vi "ReadSetting.vi"(5 "FilePath":path) -> (0 "Success":bool, 1 "Setting":T4={"TorqueSensor"={"Interface"="", "Read Unit"=enum."oz.in", "Encoder"=0, "Torque Filter"=0, "Max Torque"=0.0, "Max Power"=0.0, "Max Speed"=0.0, "Scale Factor CW"=0.0, "Scale Factor CCW"=0.0, "Scale Factor Zero"=0.0}, "TorqueSensorL"={"Interface"="", "Read Unit"=enum."Kg.cm", "Encoder"=0, "Torque Filter"=0, "Max Torque"=2.0, "Max Power"=50.0, "Max Speed"=50.0, "Scale Factor CW"=2.0, "Scale Factor CCW"=2.0, "Scale Factor Zero"=2.0}, "Power Meter"={"Wiring"=0, "Interface"="", "1P Mode"=1, "1P CurrentLimit"=0.0, "3P Mode"=1, "3P CurrentLimit"=0.0}, "Thermocouple"={"Interface"="", "value range"="T/C T type -100 ~ 400 degree C", "Channel Count"=8, "Limit 0"=0.0, "Limit 1"=0.0, "Limit 2"=0.0, "Limit 3"=0.0, "Limit 4"=0.0, "Limit 5"=0.0, "Limit 6"=0.0, "Limit 7"=0.0}, "DC-1000"={"Interface"=enum."AD-0"}, "ServoMotor"={"Interface"=enum."AD-0"}, "MotorDriver"={"D_Interface"="", "L_Interface"=""}, "TestMode"=enum."電子中軸測試", "PowerSupply"={"Interface"="", "Current"=50.0, "Voltage"=50.0}} {"Thermocouple"."Limit 7" format="%.1f"; "Thermocouple"."Limit 6" format="%.1f"; "Thermocouple"."Limit 5" format="%.1f"; "Thermocouple"."Limit 4" format="%.1f"; "Thermocouple"."Limit 3" format="%.1f"; "Thermocouple"."Limit 2" format="%.1f"; "Thermocouple"."Limit 1" format="%.1f"; "Thermocouple"."Limit 0" format="%.1f"; "Thermocouple"."Channel Count" min=0 max=24; "Power Meter"."3P Mode" items=["RMS", "MEAN", "DC"]; "Power Meter"."1P Mode" items=["RMS", "MEAN", "DC"]; "Power Meter"."Wiring" items=["AD-0", "AD-1"]; "TorqueSensorL"."Scale Factor Zero" format="%#.6f"; "TorqueSensorL"."Scale Factor CCW" format="%#.6f"; "TorqueSensorL"."Scale Factor CW" format="%#.6f"; "TorqueSensorL"."Torque Filter" items=["OFF", "10Hz", "25Hz", "50Hz", "3Hz", "2Hz", "1Hz"]; "TorqueSensorL"."Encoder" items=["60-ppr"=60, "600-ppr"=600, "6000-ppr"=6000, "8192-ppr"=8192, "20-ppr"=20, "30-ppr"=30, "1-ppr"=1, "2-ppr"=2, "6-ppr"=6]; "TorqueSensor"."Scale Factor Zero" format="%#.6f"; "TorqueSensor"."Scale Factor CCW" format="%#.6f"; "TorqueSensor"."Scale Factor CW" format="%#.6f"; "TorqueSensor"."Torque Filter" items=["OFF", "10Hz", "25Hz", "50Hz", "3Hz", "2Hz", "1Hz"]; "TorqueSensor"."Encoder" items=["60-ppr"=60, "600-ppr"=600, "6000-ppr"=6000, "8192-ppr"=8192, "20-ppr"=20, "30-ppr"=30, "1-ppr"=1, "2-ppr"=2, "6-ppr"=6]}, 2 "RcpFilePath.dup":path)   [LabVIEW 2024]
uses:
  MFActor/SystemSettings.ctl
panel:
  in  "Setting_V4":T1={"TorqueSensor"={"Interface"="", "Read Unit"=enum."Kg.cm", "Encoder"=0, "Torque Filter"=0, "Max Torque"=2.0, "Max Power"=50.0, "Max Speed"=50.0, "Scale Factor CW"=2.0, "Scale Factor CCW"=2.0, "Scale Factor Zero"=2.0}, "TorqueSensorL"={"Interface"="", "Read Unit"=enum."Kg.cm", "Encoder"=0, "Torque Filter"=0, "Max Torque"=2.0, "Max Power"=50.0, "Max Speed"=50.0, "Scale Factor CW"=2.0, "Scale Factor CCW"=2.0, "Scale Factor Zero"=2.0}, "Power Meter"={"Wiring"=0, "Interface"="", "1P Mode"=1, "1P CurrentLimit"=0.0, "3P Mode"=1, "3P CurrentLimit"=0.0}, "Thermocouple"={"Interface"="", "value range"="T/C T type -100 ~ 400 degree C", "Channel Count"=8, "Limit 0"=0.0, "Limit 1"=0.0, "Limit 2"=0.0, "Limit 3"=0.0, "Limit 4"=0.0, "Limit 5"=0.0, "Limit 6"=0.0, "Limit 7"=0.0}, "DC-1000"={"Interface"=enum."AD-1"}, "ServoMotor"={"Interface"=enum."AD-1"}, "MotorDriver"={"D_Interface"="", "L_Interface"=""}, "TestMode"=enum."電子中軸測試", "PowerSupply"={"Interface"="", "Current"=50.0, "Voltage"=50.0}} {"Thermocouple"."Limit 7" format="%.1f"; "Thermocouple"."Limit 6" format="%.1f"; "Thermocouple"."Limit 5" format="%.1f"; "Thermocouple"."Limit 4" format="%.1f"; "Thermocouple"."Limit 3" format="%.1f"; "Thermocouple"."Limit 2" format="%.1f"; "Thermocouple"."Limit 1" format="%.1f"; "Thermocouple"."Limit 0" format="%.1f"; "Thermocouple"."Channel Count" min=0 max=24; "Power Meter"."3P Mode" items=["RMS", "MEAN", "DC"]; "Power Meter"."1P Mode" items=["RMS", "MEAN", "DC"]; "Power Meter"."Wiring" items=["1P2W", "1P2W+3P3W3M"]; "TorqueSensorL"."Scale Factor Zero" format="%#.6f"; "TorqueSensorL"."Scale Factor CCW" format="%#.6f"; "TorqueSensorL"."Scale Factor CW" format="%#.6f"; "TorqueSensorL"."Torque Filter" items=["OFF", "10Hz", "25Hz", "50Hz", "3Hz", "2Hz", "1Hz"]; "TorqueSensorL"."Encoder" items=["60-ppr"=60, "600-ppr"=600, "6000-ppr"=6000, "8192-ppr"=8192, "20-ppr"=20, "30-ppr"=30, "1-ppr"=1, "2-ppr"=2, "6-ppr"=6]; "TorqueSensor"."Scale Factor Zero" format="%#.6f"; "TorqueSensor"."Scale Factor CCW" format="%#.6f"; "TorqueSensor"."Scale Factor CW" format="%#.6f"; "TorqueSensor"."Torque Filter" items=["OFF", "10Hz", "25Hz", "50Hz", "3Hz", "2Hz", "1Hz"]; "TorqueSensor"."Encoder" items=["60-ppr"=60, "600-ppr"=600, "6000-ppr"=6000, "8192-ppr"=8192, "20-ppr"=20, "30-ppr"=30, "1-ppr"=1, "2-ppr"=2, "6-ppr"=6]}
  in  "Setting_V3":T2={"TorqueSensor"={"Interface"="", "Read Unit"=enum."Kg.cm", "Encoder"=0, "Torque Filter"=0, "Max Torque"=2.0, "Max Power"=50.0, "Max Speed"=50.0, "Scale Factor CW"=2.0, "Scale Factor CCW"=2.0, "Scale Factor Zero"=2.0}, "TorqueSensorL"={"Interface"="", "Read Unit"=enum."Kg.cm", "Encoder"=0, "Torque Filter"=0, "Max Torque"=2.0, "Max Power"=50.0, "Max Speed"=50.0, "Scale Factor CW"=2.0, "Scale Factor CCW"=2.0, "Scale Factor Zero"=2.0}, "Power Meter"={"Wiring"=0, "Interface"="", "1P Mode"=1, "1P CurrentLimit"=0.0, "3P Mode"=1, "3P CurrentLimit"=0.0}, "Thermocouple"={"Interface"="", "value range"="T/C T type -100 ~ 400 degree C", "Channel Count"=8, "Limit 0"=0.0, "Limit 1"=0.0, "Limit 2"=0.0, "Limit 3"=0.0, "Limit 4"=0.0, "Limit 5"=0.0, "Limit 6"=0.0, "Limit 7"=0.0}, "DC-1000"={"Interface"=enum."AD-1"}, "ServoMotor"={"Interface"=enum."AD-1"}, "MotorDriver"={"D_Interface"="", "L_Interface"=""}, "TestMode"=enum."電子中軸測試"} {"Thermocouple"."Limit 7" format="%.1f"; "Thermocouple"."Limit 6" format="%.1f"; "Thermocouple"."Limit 5" format="%.1f"; "Thermocouple"."Limit 4" format="%.1f"; "Thermocouple"."Limit 3" format="%.1f"; "Thermocouple"."Limit 2" format="%.1f"; "Thermocouple"."Limit 1" format="%.1f"; "Thermocouple"."Limit 0" format="%.1f"; "Thermocouple"."Channel Count" min=0 max=24; "Power Meter"."3P Mode" items=["RMS", "MEAN", "DC"]; "Power Meter"."1P Mode" items=["RMS", "MEAN", "DC"]; "Power Meter"."Wiring" items=["1P2W", "1P2W+3P3W3M"]; "TorqueSensorL"."Scale Factor Zero" format="%#.6f"; "TorqueSensorL"."Scale Factor CCW" format="%#.6f"; "TorqueSensorL"."Scale Factor CW" format="%#.6f"; "TorqueSensorL"."Torque Filter" items=["OFF", "10Hz", "25Hz", "50Hz", "3Hz", "2Hz", "1Hz"]; "TorqueSensorL"."Encoder" items=["60-ppr"=60, "600-ppr"=600, "6000-ppr"=6000, "8192-ppr"=8192, "20-ppr"=20, "30-ppr"=30, "1-ppr"=1, "2-ppr"=2, "6-ppr"=6]; "TorqueSensor"."Scale Factor Zero" format="%#.6f"; "TorqueSensor"."Scale Factor CCW" format="%#.6f"; "TorqueSensor"."Scale Factor CW" format="%#.6f"; "TorqueSensor"."Torque Filter" items=["OFF", "10Hz", "25Hz", "50Hz", "3Hz", "2Hz", "1Hz"]; "TorqueSensor"."Encoder" items=["60-ppr"=60, "600-ppr"=600, "6000-ppr"=6000, "8192-ppr"=8192, "20-ppr"=20, "30-ppr"=30, "1-ppr"=1, "2-ppr"=2, "6-ppr"=6]}
  in  "Setting_V2":T3={"TorqueSensor"={"Interface"="", "Read Unit"=enum."Kg.cm", "Encoder"=0, "Torque Filter"=0, "Max Torque"=2.0, "Max Power"=50.0, "Max Speed"=50.0, "Scale Factor CW"=2.0, "Scale Factor CCW"=2.0, "Scale Factor Zero"=2.0}, "DC-1000"={"Interface"=enum."AD-1"}, "ServoMotor"={"Interface"=enum."AD-1"}, "MotorDriver"={"D_Interface"="", "L_Interface"=""}, "SwapDL"=FALSE} {"TorqueSensor"."Scale Factor Zero" format="%#.6f"; "TorqueSensor"."Scale Factor CCW" format="%#.6f"; "TorqueSensor"."Scale Factor CW" format="%#.6f"; "TorqueSensor"."Torque Filter" items=["OFF", "10Hz", "25Hz", "50Hz", "3Hz", "2Hz", "1Hz"]; "TorqueSensor"."Encoder" items=["60-ppr"=60, "600-ppr"=600, "6000-ppr"=6000, "8192-ppr"=8192, "20-ppr"=20, "30-ppr"=30, "1-ppr"=1, "2-ppr"=2, "6-ppr"=6]}
  in  "Setting_V1":T5={"TorqueSensor"={"Interface"="", "Read Unit"=enum."Kg.cm", "Encoder"=0, "Torque Filter"=0, "Max Torque"=2.0, "Max Power"=50.0, "Max Speed"=50.0, "Scale Factor CW"=2.0, "Scale Factor CCW"=2.0, "Scale Factor Zero"=2.0}, "DC-1000"={"Interface"=enum."AD-1"}, "ServoMotor"={"Interface"=enum."AD-1"}, "MotorDriver"={"D_Interface"="", "L_Interface"=""}} {"TorqueSensor"."Scale Factor Zero" format="%#.6f"; "TorqueSensor"."Scale Factor CCW" format="%#.6f"; "TorqueSensor"."Scale Factor CW" format="%#.6f"; "TorqueSensor"."Torque Filter" items=["OFF", "10Hz", "25Hz", "50Hz", "3Hz", "2Hz", "1Hz"]; "TorqueSensor"."Encoder" items=["60-ppr"=60, "600-ppr"=600, "6000-ppr"=6000, "8192-ppr"=8192, "20-ppr"=20, "30-ppr"=30, "1-ppr"=1, "2-ppr"=2, "6-ppr"=6]}
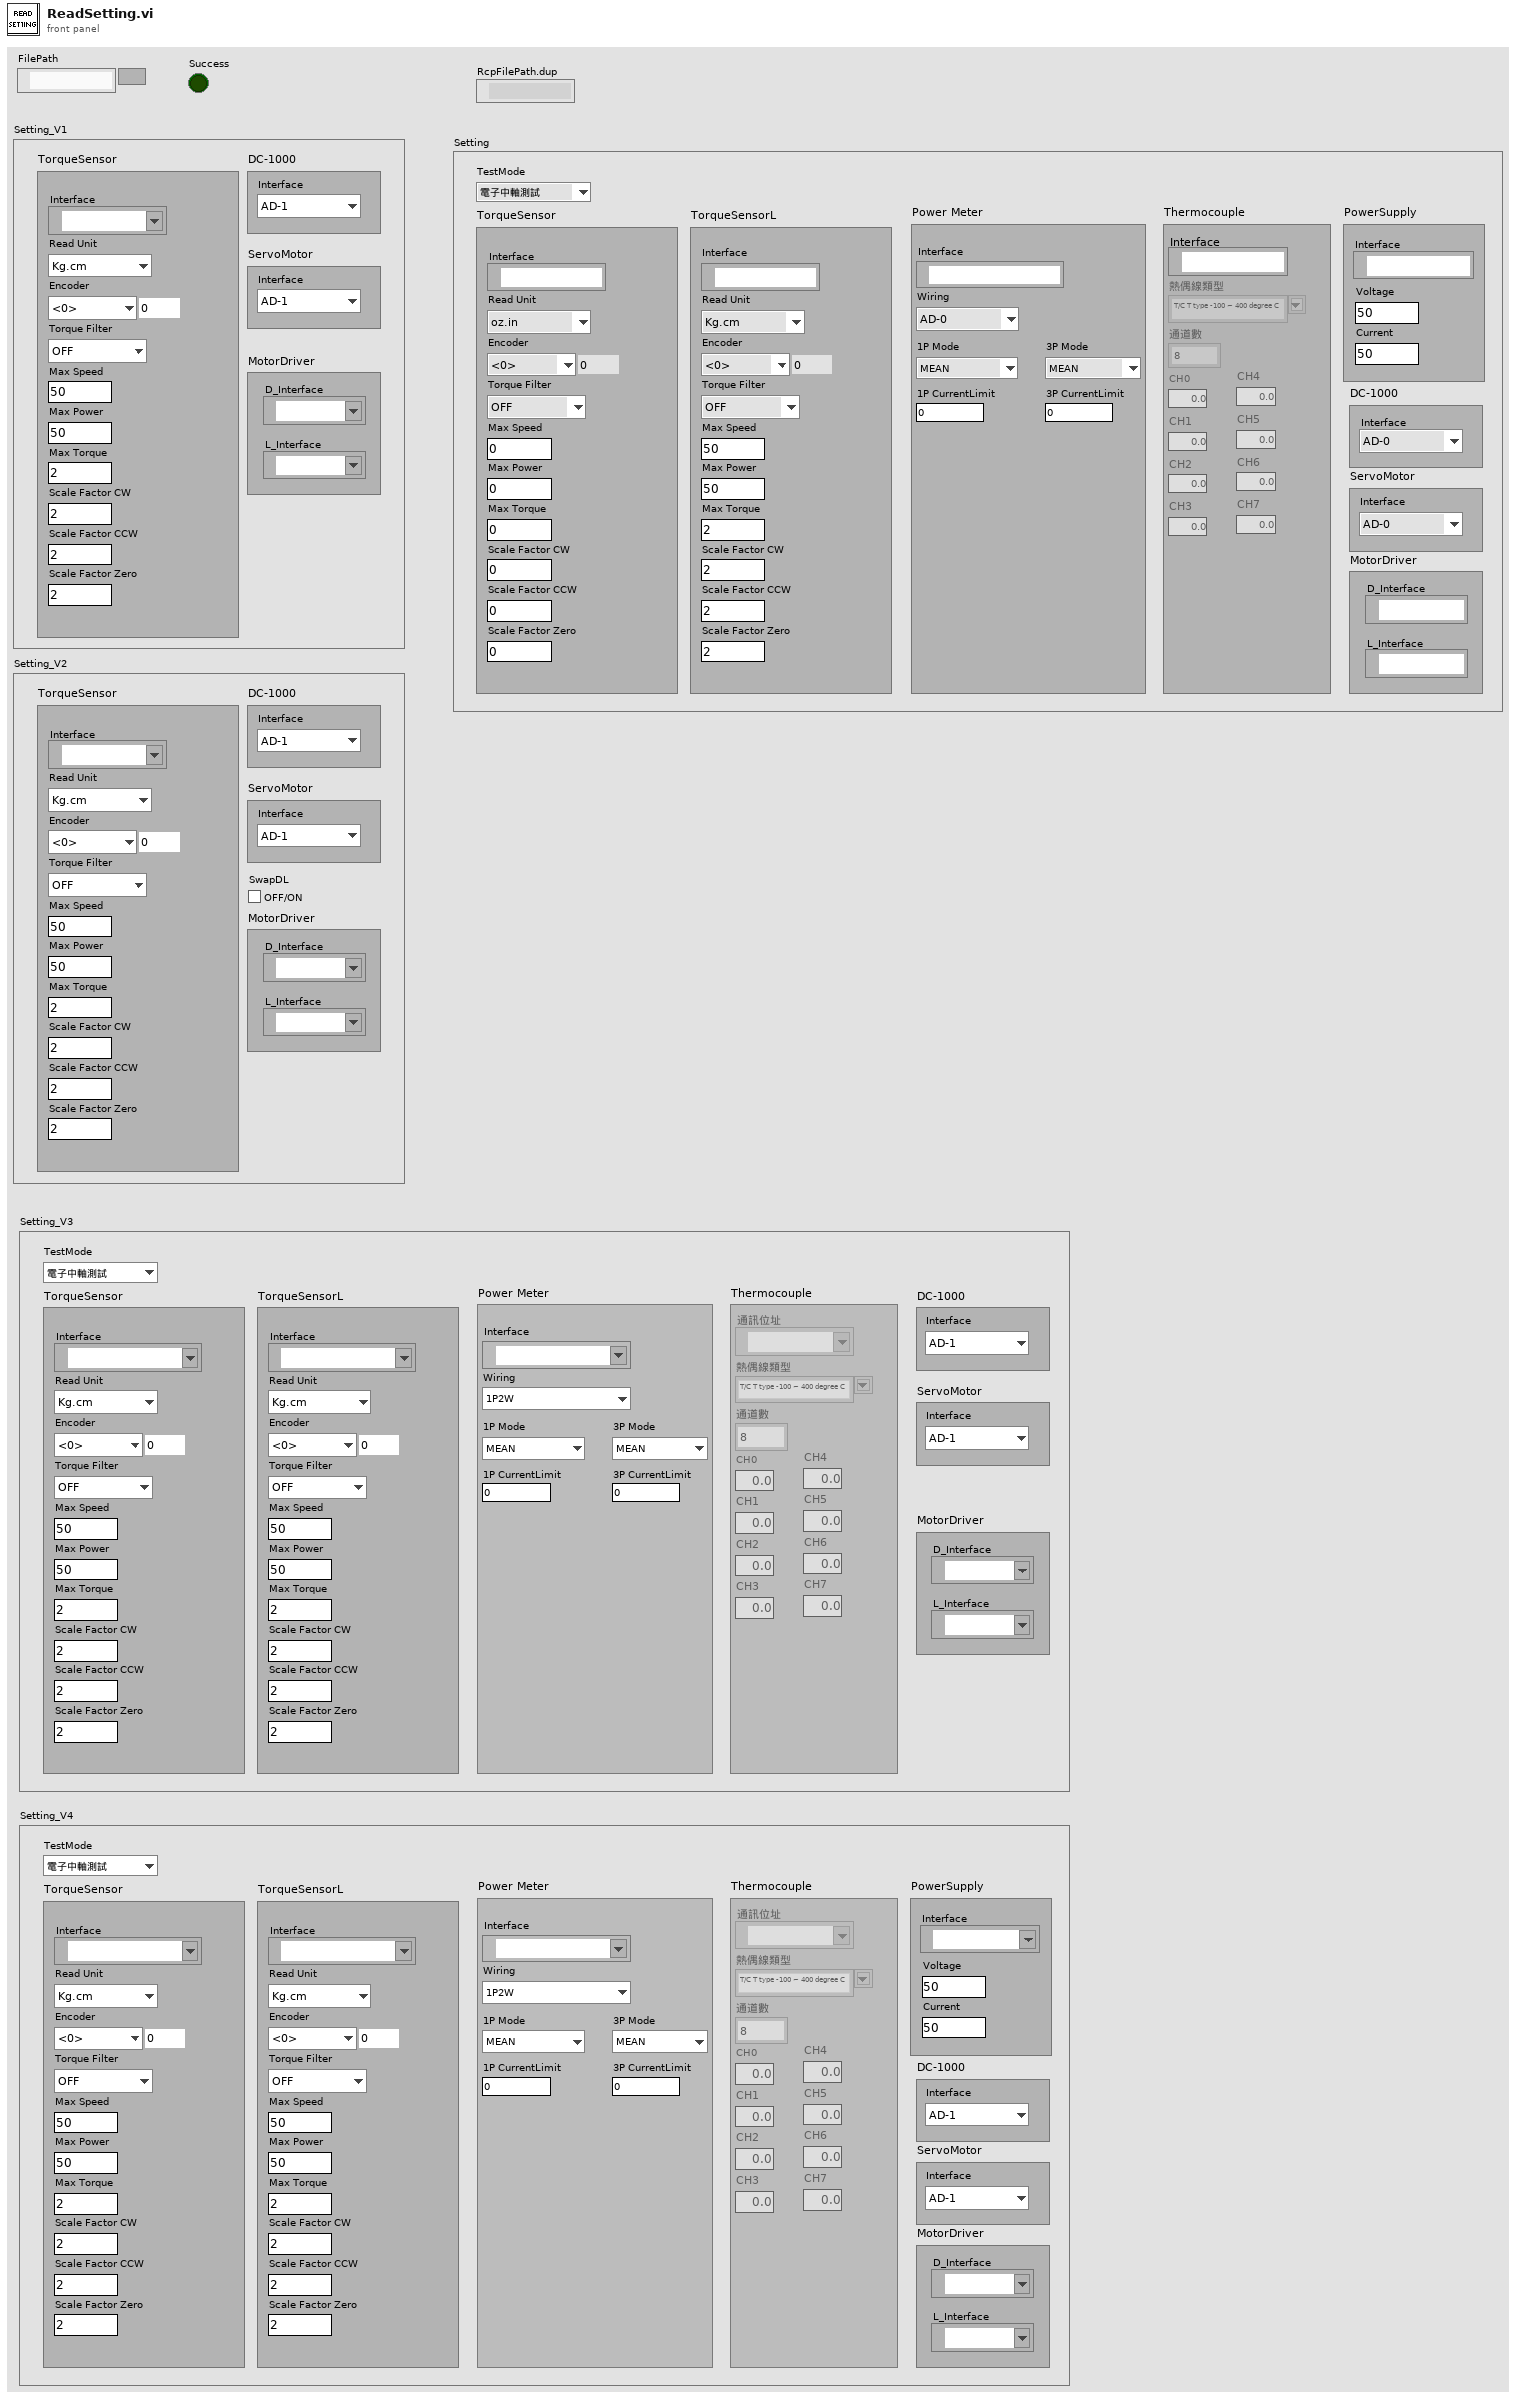
[diagram p1: front panel]
types:
  T1 = cluster{"TorqueSensor":cluster{"Interface":refnum<visa-resource-name>, "Read Unit":enum16{"oz.in", "oz.ft", "lb.in", "lb.ft", "g.cm", "Kg.cm", "mN.m", "cN.m", "N.m"}, "Encoder":u16, "Torque Filter":u16, "Max Torque":dbl, "Max Power":dbl, "Max Speed":dbl, "Scale Factor CW":dbl, "Scale Factor CCW":dbl, "Scale Factor Zero":dbl}, "TorqueSensorL":cluster{"Interface":refnum<visa-resource-name>, "Read Unit":enum16{"oz.in", "oz.ft", "lb.in", "lb.ft", "g.cm", "Kg.cm", "mN.m", "cN.m", "N.m"}, "Encoder":u16, "Torque Filter":u16, "Max Torque":dbl, "Max Power":dbl, "Max Speed":dbl, "Scale Factor CW":dbl, "Scale Factor CCW":dbl, "Scale Factor Zero":dbl}, "Power Meter":cluster{"Wiring":u16, "Interface":refnum<visa-resource-name>, "1P Mode":u16, "1P CurrentLimit":dbl, "3P Mode":u16, "3P CurrentLimit":dbl}, "Thermocouple":cluster{"Interface":refnum<visa-resource-name>, "value range":string, "Channel Count":i32, "Limit 0":dbl, "Limit 1":dbl, "Limit 2":dbl, "Limit 3":dbl, "Limit 4":dbl, "Limit 5":dbl, "Limit 6":dbl, "Limit 7":dbl}, "DC-1000":cluster{"Interface":enum16{"AD-0", "AD-1"}}, "ServoMotor":cluster{"Interface":enum16{"AD-0", "AD-1"}}, "MotorDriver":cluster{"D_Interface":refnum<visa-resource-name>, "L_Interface":refnum<visa-resource-name>}, "TestMode":enum16{"電子中軸測試", "中置電機測試"}, "PowerSupply":cluster{"Interface":refnum<visa-resource-name>, "Current":dbl, "Voltage":dbl}}
  T2 = cluster{"TorqueSensor":cluster{"Interface":refnum<visa-resource-name>, "Read Unit":enum16{"oz.in", "oz.ft", "lb.in", "lb.ft", "g.cm", "Kg.cm", "mN.m", "cN.m", "N.m"}, "Encoder":u16, "Torque Filter":u16, "Max Torque":dbl, "Max Power":dbl, "Max Speed":dbl, "Scale Factor CW":dbl, "Scale Factor CCW":dbl, "Scale Factor Zero":dbl}, "TorqueSensorL":cluster{"Interface":refnum<visa-resource-name>, "Read Unit":enum16{"oz.in", "oz.ft", "lb.in", "lb.ft", "g.cm", "Kg.cm", "mN.m", "cN.m", "N.m"}, "Encoder":u16, "Torque Filter":u16, "Max Torque":dbl, "Max Power":dbl, "Max Speed":dbl, "Scale Factor CW":dbl, "Scale Factor CCW":dbl, "Scale Factor Zero":dbl}, "Power Meter":cluster{"Wiring":u16, "Interface":refnum<visa-resource-name>, "1P Mode":u16, "1P CurrentLimit":dbl, "3P Mode":u16, "3P CurrentLimit":dbl}, "Thermocouple":cluster{"Interface":refnum<visa-resource-name>, "value range":string, "Channel Count":i32, "Limit 0":dbl, "Limit 1":dbl, "Limit 2":dbl, "Limit 3":dbl, "Limit 4":dbl, "Limit 5":dbl, "Limit 6":dbl, "Limit 7":dbl}, "DC-1000":cluster{"Interface":enum16{"AD-0", "AD-1"}}, "ServoMotor":cluster{"Interface":enum16{"AD-0", "AD-1"}}, "MotorDriver":cluster{"D_Interface":refnum<visa-resource-name>, "L_Interface":refnum<visa-resource-name>}, "TestMode":enum16{"電子中軸測試", "中置電機測試"}}
  T3 = cluster{"TorqueSensor":cluster{"Interface":refnum<visa-resource-name>, "Read Unit":enum16{"oz.in", "oz.ft", "lb.in", "lb.ft", "g.cm", "Kg.cm", "mN.m", "cN.m", "N.m"}, "Encoder":u16, "Torque Filter":u16, "Max Torque":dbl, "Max Power":dbl, "Max Speed":dbl, "Scale Factor CW":dbl, "Scale Factor CCW":dbl, "Scale Factor Zero":dbl}, "DC-1000":cluster{"Interface":enum16{"AD-0", "AD-1"}}, "ServoMotor":cluster{"Interface":enum16{"AD-0", "AD-1"}}, "MotorDriver":cluster{"D_Interface":refnum<visa-resource-name>, "L_Interface":refnum<visa-resource-name>}, "SwapDL":bool}
  T4 = typedef "SystemSettings.ctl" = cluster{"TorqueSensor":cluster{"Interface":refnum<visa-resource-name>, "Read Unit":enum16{"oz.in", "oz.ft", "lb.in", "lb.ft", "g.cm", "Kg.cm", "mN.m", "cN.m", "N.m"}, "Encoder":u16, "Torque Filter":u16, "Max Torque":dbl, "Max Power":dbl, "Max Speed":dbl, "Scale Factor CW":dbl, "Scale Factor CCW":dbl, "Scale Factor Zero":dbl}, "TorqueSensorL":cluster{"Interface":refnum<visa-resource-name>, "Read Unit":enum16{"oz.in", "oz.ft", "lb.in", "lb.ft", "g.cm", "Kg.cm", "mN.m", "cN.m", "N.m"}, "Encoder":u16, "Torque Filter":u16, "Max Torque":dbl, "Max Power":dbl, "Max Speed":dbl, "Scale Factor CW":dbl, "Scale Factor CCW":dbl, "Scale Factor Zero":dbl}, "Power Meter":cluster{"Wiring":u16, "Interface":refnum<visa-resource-name>, "1P Mode":u16, "1P CurrentLimit":dbl, "3P Mode":u16, "3P CurrentLimit":dbl}, "Thermocouple":cluster{"Interface":refnum<visa-resource-name>, "value range":string, "Channel Count":i32, "Limit 0":dbl, "Limit 1":dbl, "Limit 2":dbl, "Limit 3":dbl, "Limit 4":dbl, "Limit 5":dbl, "Limit 6":dbl, "Limit 7":dbl}, "DC-1000":cluster{"Interface":enum16{"AD-0", "AD-1"}}, "ServoMotor":cluster{"Interface":enum16{"AD-0", "AD-1"}}, "MotorDriver":cluster{"D_Interface":refnum<visa-resource-name>, "L_Interface":refnum<visa-resource-name>}, "TestMode":enum16{"電子中軸測試", "中置電機測試"}, "PowerSupply":cluster{"Interface":refnum<visa-resource-name>, "Current":dbl, "Voltage":dbl}}
  T5 = cluster{"TorqueSensor":cluster{"Interface":refnum<visa-resource-name>, "Read Unit":enum16{"oz.in", "oz.ft", "lb.in", "lb.ft", "g.cm", "Kg.cm", "mN.m", "cN.m", "N.m"}, "Encoder":u16, "Torque Filter":u16, "Max Torque":dbl, "Max Power":dbl, "Max Speed":dbl, "Scale Factor CW":dbl, "Scale Factor CCW":dbl, "Scale Factor Zero":dbl}, "DC-1000":cluster{"Interface":enum16{"AD-0", "AD-1"}}, "ServoMotor":cluster{"Interface":enum16{"AD-0", "AD-1"}}, "MotorDriver":cluster{"D_Interface":refnum<visa-resource-name>, "L_Interface":refnum<visa-resource-name>}}
  T6 = enum16{"open", "replace", "create", "open or create", "replace or create", "replace or create with confirmation"}
  T7 = cluster{"Interface":refnum<visa-resource-name>, "Current":dbl, "Voltage":dbl}
  T8 = cluster{"Interface":refnum<visa-resource-name>, "value range":string, "Channel Count":i32, "Limit 0":dbl, "Limit 1":dbl, "Limit 2":dbl, "Limit 3":dbl, "Limit 4":dbl, "Limit 5":dbl, "Limit 6":dbl, "Limit 7":dbl}
  T9 = cluster{"Wiring":u16, "Interface":refnum<visa-resource-name>, "1P Mode":u16, "1P CurrentLimit":dbl, "3P Mode":u16, "3P CurrentLimit":dbl}
  T10 = cluster{"Interface":refnum<visa-resource-name>, "Read Unit":enum16{"oz.in", "oz.ft", "lb.in", "lb.ft", "g.cm", "Kg.cm", "mN.m", "cN.m", "N.m"}, "Encoder":u16, "Torque Filter":u16, "Max Torque":dbl, "Max Power":dbl, "Max Speed":dbl, "Scale Factor CW":dbl, "Scale Factor CCW":dbl, "Scale Factor Zero":dbl}
  T11 = cluster{"D_Interface":refnum<visa-resource-name>, "L_Interface":refnum<visa-resource-name>}
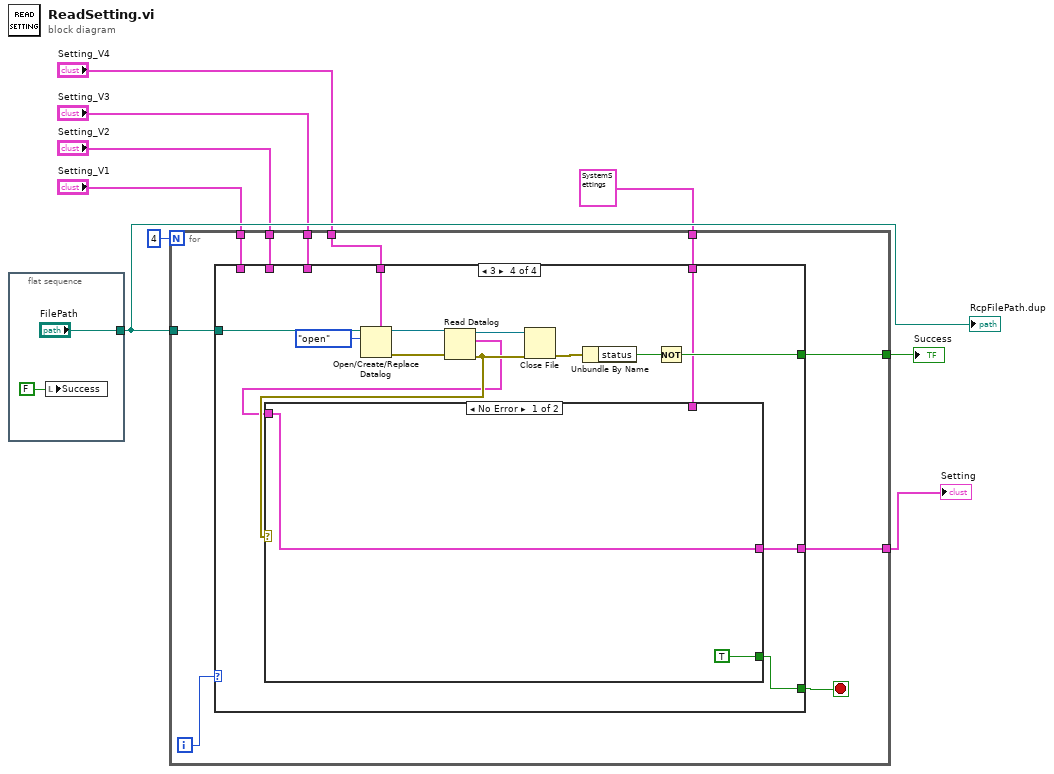
[diagram p0: block diagram]
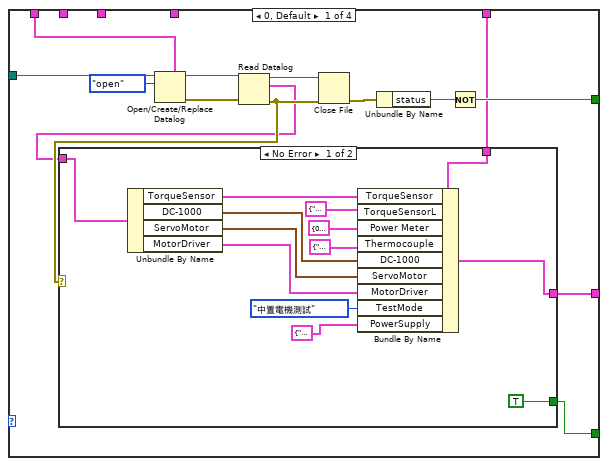
[diagram p2: hidden frame]
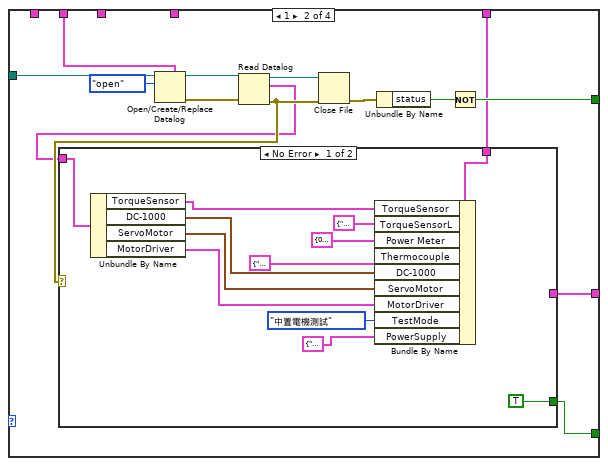
[diagram p4: hidden frame]
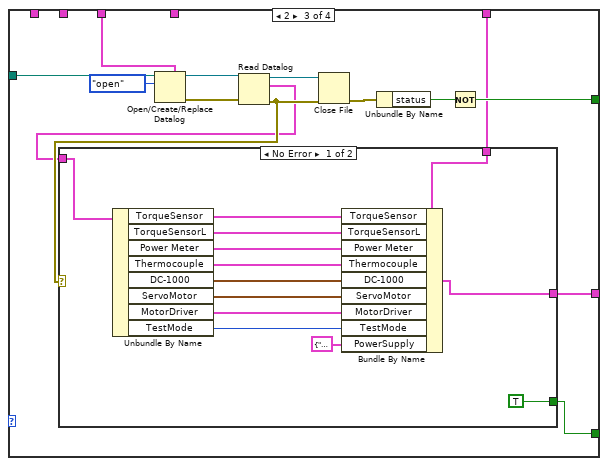
[diagram p6: hidden frame]
diagram:
  n1 = flat-sequence {
    tunnel: ["FilePath"] -> w8
    frame #0 {
      n2 = local write "Success"(FALSE ("Success")) -> ()
    }
  }
  n3 = for {
    N: 4 -> [_]
    tunnel: w8 -> [w21]
    tunnel: "Setting_V1" -> [w20]
    tunnel: [w18] -> w7
    tunnel: T4 {"TorqueSensor"={"Interface"="", "Read Unit"=enum."oz.in", "Encoder"=0, "Torque Filter"=0, "Max Torque"=0.0, "Max Power"=0.0, "Max Speed"=0.0, "Scale Factor CW"=0.0, "Scale Factor CCW"=0.0, "Scale Factor Zero"=0.0}, "TorqueSensorL"={"Interface"="", "Read Unit"=enum."Kg.cm", "Encoder"=0, "Torque Filter"=0, "Max Torque"=2.0, "Max Power"=50.0, "Max Speed"=50.0, "Scale Factor CW"=2.0, "Scale Factor CCW"=2.0, "Scale Factor Zero"=2.0}, "Power Meter"={"Wiring"=0, "Interface"="", "1P Mode"=1, "1P CurrentLimit"=0.0, "3P Mode"=1, "3P CurrentLimit"=0.0}, "Thermocouple"={"Interface"="", "value range"="T/C T type -100 ~ 400 degree C", "Channel Count"=8, "Limit 0"=0.0, "Limit 1"=0.0, "Limit 2"=0.0, "Limit 3"=0.0, "Limit 4"=0.0, "Limit 5"=0.0, "Limit 6"=0.0, "Limit 7"=0.0}, "DC-1000"={"Interface"=enum."AD-0"}, "ServoMotor"={"Interface"=enum."AD-0"}, "MotorDriver"={"D_Interface"="", "L_Interface"=""}, "TestMode"=enum."電子中軸測試", "PowerSupply"={"Interface"="", "Current"=50.0, "Voltage"=50.0}} ("Setting") -> [w17]
    tunnel: [w16] -> w5
    tunnel: "Setting_V2" -> [w14]
    tunnel: "Setting_V3" -> [w13]
    tunnel: "Setting_V4" -> [w12]
    i -> [w15]
    stop <- w19 stop-if-true
    n4 = case shown="3" w15 {
      tunnel: w21 -> [w31 w59 w86 w114]
      tunnel: w20 -> [w30 _ _ _]
      tunnel: [w29 w58 w85 w113] -> w19
      tunnel: [w26 w55 w82 w110] -> w18
      tunnel: w17 -> [w23 w52 w79 w107]
      tunnel: [w22 w51 w78 w106] -> w16
      tunnel: w14 -> [_ w50 _ _]
      tunnel: w13 -> [_ _ w77 _]
      tunnel: w12 -> [_ _ _ w105]
      frame 0, Default {
        n5 = Open/Create/Replace Datalog(5:w30, 10:T6."open" ("operation (0:open)"), 11:w31) -> (0:w34:errorcluster, 3:w33:refnum<k1>)  [unwired: 3 in, 1 out]
        n6 = Read Datalog(4:w34, 7:w33) -> (0:w25:errorcluster, 2:w24:T5, 3:w35:refnum<k1>)  [unwired: 1 in]
        n7 = case shown="No Error" w25 {
          tunnel: [TRUE _] -> w29
          tunnel: w24 -> [w47 _]
          tunnel: w23 -> [w46 w49]
          tunnel: [w45 w49] -> w22
          frame No Error {
            n8 = Unbundle By Name(w47) -> ("TorqueSensor"=w44:T10, "DC-1000"=w40:cluster{"Interface":enum16{"AD-0", "AD-1"}}, "ServoMotor"=w39:cluster{"Interface":enum16{"AD-0", "AD-1"}}, "MotorDriver"=w38:T11)
            n9 = Bundle By Name(cluster=w46, "TorqueSensor"=w44, "TorqueSensorL"=T10 {"Interface"="", "Read Unit"=enum."oz.in", "Encoder"=0, "Torque Filter"=0, "Max Torque"=0.0, "Max Power"=0.0, "Max Speed"=0.0, "Scale Factor CW"=0.0, "Scale Factor CCW"=0.0, "Scale Factor Zero"=0.0}, "Power Meter"=T9 {"Wiring"=0, "Interface"="", "1P Mode"=0, "1P CurrentLimit"=0.0, "3P Mode"=0, "3P CurrentLimit"=0.0}, "Thermocouple"=T8 {"Interface"="", "value range"="", "Channel Count"=0, "Limit 0"=0.0, "Limit 1"=0.0, "Limit 2"=0.0, "Limit 3"=0.0, "Limit 4"=0.0, "Limit 5"=0.0, "Limit 6"=0.0, "Limit 7"=0.0}, "DC-1000"=w40, "ServoMotor"=w39, "MotorDriver"=w38, "TestMode"=enum16{"電子中軸測試", "中置電機測試"}."中置電機測試", "PowerSupply"=T7 {"Interface"="", "Current"=0.0, "Voltage"=0.0}) -> (w45:T4)
          }
          frame Error {
          }
        }
        n10 = Close File(refnum=w35, error in=w25) -> (error out=w28:errorcluster)  [unwired: 1 out]
        n11 = Unbundle By Name(w28) -> ("status"=w27:bool)
        n12 = Not(x=w27) -> (.not. x?=w26:bool)
      }
      frame 1 {
        n13 = Open/Create/Replace Datalog(5:w50, 10:T6."open" ("operation (0:open)"), 11:w59) -> (0:w62:errorcluster, 3:w61:refnum<k1>)  [unwired: 3 in, 1 out]
        n14 = Read Datalog(4:w62, 7:w61) -> (0:w54:errorcluster, 2:w53:T3, 3:w63:refnum<k1>)  [unwired: 1 in]
        n15 = case shown="No Error" w54 {
          tunnel: [TRUE _] -> w58
          tunnel: w53 -> [w74 _]
          tunnel: w52 -> [w73 w76]
          tunnel: [_ w76] -> w51
          frame No Error {
            n16 = Unbundle By Name(w74) -> ("TorqueSensor"=w72:T10, "DC-1000"=w71:cluster{"Interface":enum16{"AD-0", "AD-1"}}, "ServoMotor"=w70:cluster{"Interface":enum16{"AD-0", "AD-1"}}, "MotorDriver"=w69:T11)
            n17 = Bundle By Name(cluster=w73, "TorqueSensor"=w72, "TorqueSensorL"=T10 {"Interface"="", "Read Unit"=enum."oz.in", "Encoder"=0, "Torque Filter"=0, "Max Torque"=0.0, "Max Power"=0.0, "Max Speed"=0.0, "Scale Factor CW"=0.0, "Scale Factor CCW"=0.0, "Scale Factor Zero"=0.0}, "Power Meter"=T9 {"Wiring"=0, "Interface"="", "1P Mode"=0, "1P CurrentLimit"=0.0, "3P Mode"=0, "3P CurrentLimit"=0.0}, "Thermocouple"=T8 {"Interface"="", "value range"="", "Channel Count"=0, "Limit 0"=0.0, "Limit 1"=0.0, "Limit 2"=0.0, "Limit 3"=0.0, "Limit 4"=0.0, "Limit 5"=0.0, "Limit 6"=0.0, "Limit 7"=0.0}, "DC-1000"=w71, "ServoMotor"=w70, "MotorDriver"=w69, "TestMode"=enum16{"電子中軸測試", "中置電機測試"}."中置電機測試", "PowerSupply"=T7 {"Interface"="", "Current"=0.0, "Voltage"=0.0}) -> ()  [unwired: 1 out]
          }
          frame Error {
          }
        }
        n18 = Close File(refnum=w63, error in=w54) -> (error out=w57:errorcluster)  [unwired: 1 out]
        n19 = Unbundle By Name(w57) -> ("status"=w56:bool)
        n20 = Not(x=w56) -> (.not. x?=w55:bool)
      }
      frame 2 {
        n21 = Open/Create/Replace Datalog(5:w77, 10:T6."open" ("operation (0:open)"), 11:w86) -> (0:w89:errorcluster, 3:w88:refnum<k1>)  [unwired: 3 in, 1 out]
        n22 = Read Datalog(4:w89, 7:w88) -> (0:w81:errorcluster, 2:w80:T2, 3:w90:refnum<k1>)  [unwired: 1 in]
        n23 = case shown="No Error" w81 {
          tunnel: [TRUE _] -> w85
          tunnel: w80 -> [w102 _]
          tunnel: w79 -> [w101 w104]
          tunnel: [w91 w104] -> w78
          frame No Error {
            n24 = Unbundle By Name(w102) -> ("TorqueSensor"=w100:T10, "TorqueSensorL"=w99:T10, "Power Meter"=w98:T9, "Thermocouple"=w97:T8, "DC-1000"=w96:cluster{"Interface":enum16{"AD-0", "AD-1"}}, "ServoMotor"=w95:cluster{"Interface":enum16{"AD-0", "AD-1"}}, "MotorDriver"=w94:T11, "TestMode"=w93:enum16{"電子中軸測試", "中置電機測試"})
            n25 = Bundle By Name(cluster=w101, "TorqueSensor"=w100, "TorqueSensorL"=w99, "Power Meter"=w98, "Thermocouple"=w97, "DC-1000"=w96, "ServoMotor"=w95, "MotorDriver"=w94, "TestMode"=w93, "PowerSupply"=T7 {"Interface"="", "Current"=0.0, "Voltage"=0.0}) -> (w91:T4)
          }
          frame Error {
          }
        }
        n26 = Close File(refnum=w90, error in=w81) -> (error out=w84:errorcluster)  [unwired: 1 out]
        n27 = Unbundle By Name(w84) -> ("status"=w83:bool)
        n28 = Not(x=w83) -> (.not. x?=w82:bool)
      }
      frame 3 {
        n29 = Open/Create/Replace Datalog(5:w105, 10:T6."open" ("operation (0:open)"), 11:w114) -> (0:w117:errorcluster, 3:w116:refnum<k1>)  [unwired: 3 in, 1 out]
        n30 = Read Datalog(4:w117, 7:w116) -> (0:w109:errorcluster, 2:w108:T1, 3:w118:refnum<k1>)  [unwired: 1 in]
        n31 = case shown="No Error" w109 {
          tunnel: [TRUE _] -> w113
          tunnel: w108 -> [w119 _]
          tunnel: w107 -> [_ w121]
          tunnel: [w119 w121] -> w106
          frame No Error {
          }
          frame Error {
          }
        }
        n32 = Close File(refnum=w118, error in=w109) -> (error out=w112:errorcluster)  [unwired: 1 out]
        n33 = Unbundle By Name(w112) -> ("status"=w111:bool)
        n34 = Not(x=w111) -> (.not. x?=w110:bool)
      }
    }
  }
  "Success" <- w7
  "Setting" <- w5
  "RcpFilePath.dup" <- w8
